vi "Send_Email_Async.vi"   [LabVIEW 2010]
uses:
  Email_transfer_global.vi
types:
  T1 = cluster{"path":path, "data":string, "binary":bool, "MIME content-type \n(application/octet-stream)":string}[]
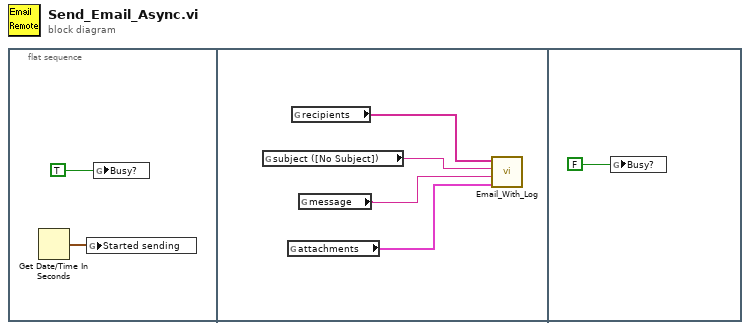
[diagram p0: block diagram]
diagram:
  n1 = flat-sequence {
    frame #0 {
      n2 = Get Date/Time In Seconds() -> (seconds since 1Jan1904=w1:timestamp)
      n3 = global write "Email_transfer_global.vi" "Started sending"(w1) -> ()
      n4 = global write "Email_transfer_global.vi" "Busy?"(TRUE ("Busy?")) -> ()
    }
    frame #1 {
      n5 = global read "Email_transfer_global.vi" "subject ([No Subject])"() -> (w5:string)
      n6 = global read "Email_transfer_global.vi" "attachments"() -> (w3:T1)
      n7 = global read "Email_transfer_global.vi" "recipients"() -> (w6:string[])
      n8 = global read "Email_transfer_global.vi" "message"() -> (w4:string)
      n9 = call "Email_With_Log.vi"("recipients"=w6, "subject ([No Subject])"=w5, "message"=w4, "attachments"=w3) -> ()  [unwired: 3 out]
    }
    frame #2 {
      n10 = global write "Email_transfer_global.vi" "Busy?"(FALSE ("Busy?")) -> ()
    }
  }
